vi "GV preframegate.vi"() -> ()   [LabVIEW 2017]
panel:
  out "Preframegate":bool
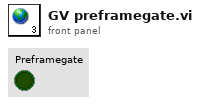
[diagram p1: front panel]
diagram:
